vi "Approach_VUW.vi"(7 "Computer called (T/F)":bool) -> ()   [LabVIEW 2023]
uses:
  Sub_Vi/TypeDefsControls/Zposition.ctl
  Sub_Vi/TypeDefsControls/Piezo Velocity.ctl
  Sub_Vi/TypeDefsControls/Voltage.ctl
  Sub_Vi/TypeDefsControls/Xposition.ctl
  Sub_Vi/TypeDefsControls/Yposition.ctl
  Sub_Vi/TypeDefs/WayPointCluster.ctl
  Sub_Vi/TypeDefs/ChangeOnFly.ctl
  Sub_Vi/TypeDefs/Settings.ctl
  Sub_Vi/TypeDefs/Display.ctl
  Sub_Vi/TypeDefsControls/Feedback Type.ctl
  Settings.vi
panel:
  out "Current 1":cluster{"Y":dbl[], "Y":dbl[]}[](graph)
  in  "Boolean Negative":bool
  in  "Boolean Positive":bool=TRUE
  in  "Feedback Threshold (A)\nUpper":dbl
  in  "Feedback Type":T1=enum."Current 1"
  in  "Display Cluster":T2
  in  "SettingsCluster":T3={"Sample Rate (us)"=1, "Samples Per Data Point (int, power of 2)"=1000, "DistanceToBulk (um)"=-1.0, "HoldTimeScaler"=1, "SaveData"=TRUE, "DistanceToBulk (um) 2"=-1.0, "DistanceToBulk (um) 3"=-1.0}
  in  "ChangeonFly":T4
  in  "WayPointCluster":T5
  in  "Start scan Button":bool
  in  "Stop":bool
  in  "Pause":bool
  in  "Feedback Threshold (A)\nLower":dbl
  in  "Set X":bool
  in  "Set Y":bool
  in  "Y":T6=100.0 min=0.0 max=100000.0
  in  "X":T7=100.0 min=0.0 max=100000.0
  in  "Approach Voltage (V)":T8 min=-10.0 max=10.0
  in  "Approach Rate (µm/s)":T9=0.1 min=0.0
  in  "End Extension (µm)":T10 min=0.0 max=100000.0
  in  "Start Extention (µm)":T10=150.0 min=0.0 max=100000.0
  out "?":cluster{"Y":dbl[], "Y":dbl[]}[](graph)
  out "?":dbl[](graph)
  # "Settings"
  # "Pause at"
  # "Advanced Settings"
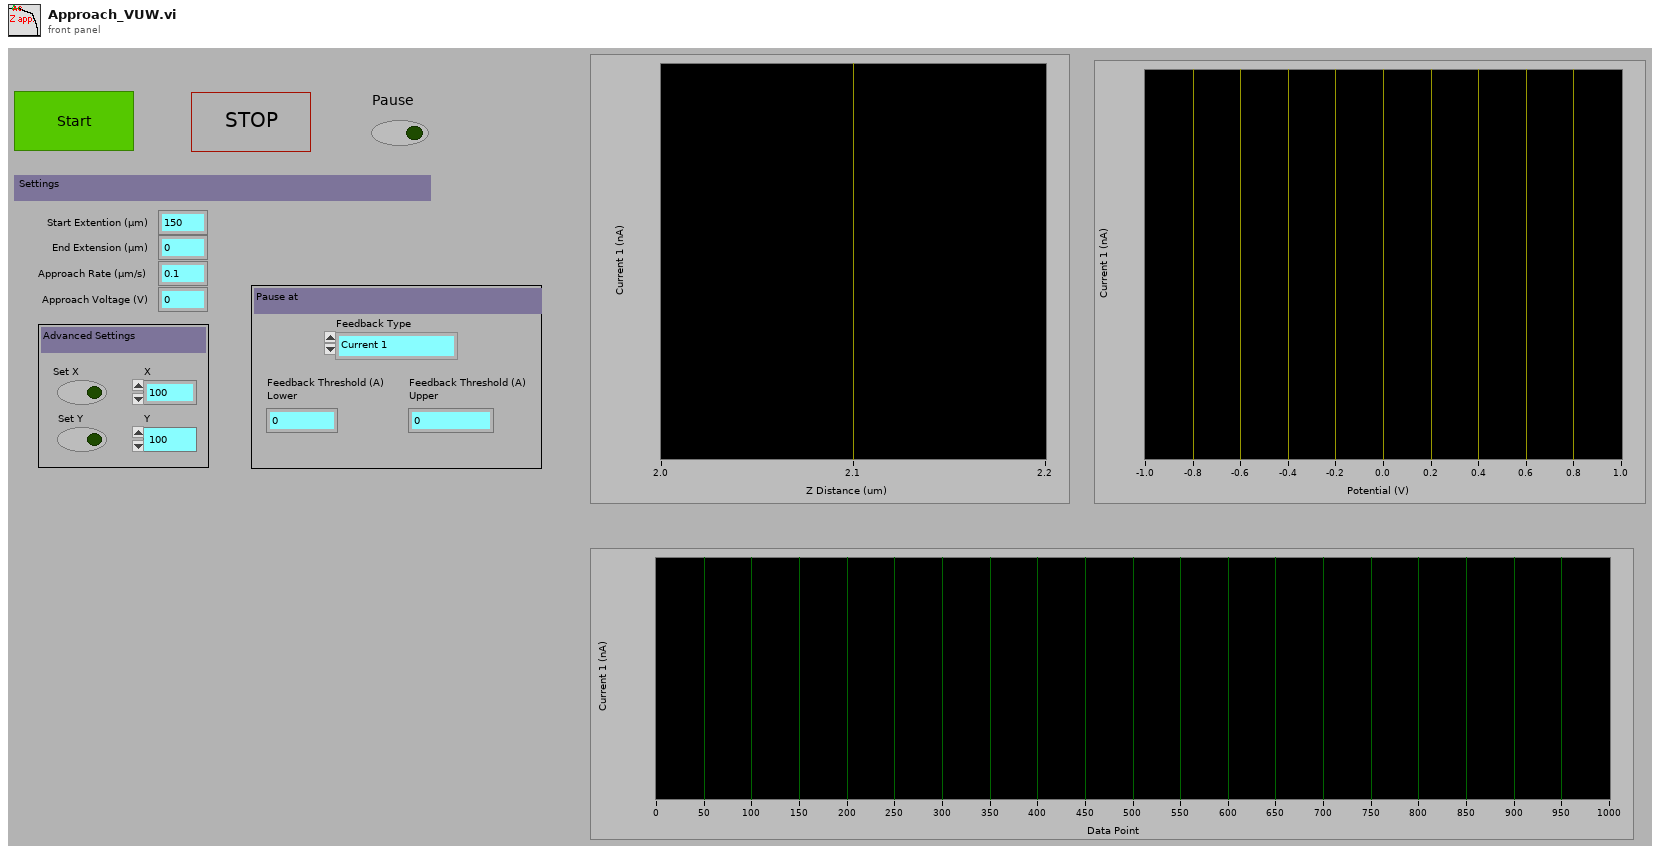
[diagram p1: front panel]
types:
  T1 = typedef "Feedback Type.ctl" = enum16{"AC Magnitude", "Current 1", "Current 2", "Phase"}
  T2 = typedef "Display.ctl" = cluster{"X":refnum<vi>, "Y":refnum<vi>, "Z":refnum<vi>, "Amp":refnum<vi>, "Phase":refnum<vi>, "t vs Z":refnum<vi>, "t vs C1":refnum<vi>, "t vs C2":refnum<vi>, "t vs C3":refnum<vi>, "t vs Amp":refnum<vi>, "t vs Phase":refnum<vi>, "t vs X":refnum<vi>, "t vs Y":refnum<vi>, "Z vs C1":refnum<vi>, "Z vs C2":refnum<vi>, "Z vs C3":refnum<vi>, "V vs C1":refnum<vi>, "V vs C2":refnum<vi>, "V vs C3":refnum<vi>, "X/Y/Z F":refnum<vi>, "X/Y/Z R":refnum<vi>, "X/Y/C1 F":refnum<vi>, "X/Y/C1 R":refnum<vi>, "X/Y/C2 F":refnum<vi>, "X/Y/C2 R":refnum<vi>, "X/Y/C3 F":refnum<vi>, "X/Y/C3 R":refnum<vi>, "NumberOfLines":u16, "um Per Pixel":dbl, "um Per Line":dbl, "X Center":dbl, "Hop X/Y/Z":refnum<vi>, "Hop X/Y/C1":refnum<vi>, "Hop X/Y/C2":refnum<vi>, "Hop X/Y/C3":refnum<vi>, "X Width":dbl, "Y Width":dbl, "Hopping Distance":dbl, "V2 vs C1":refnum<vi>, "V vs Phase":refnum<vi>, "Y Center":dbl, "Number of Pixels":dbl, "V2 vs C2":refnum<vi>, "V2 vs C3":refnum<vi>, "V vs y":refnum<vi>, "V2 vs y":refnum<vi>, "Z vs Amp":refnum<vi>, "Z vs Phase":refnum<vi>}
  T3 = typedef "Settings.ctl" = cluster{"Sample Rate (us)":u32, "Samples Per Data Point (int, power of 2)":i16, "DistanceToBulk (um)":dbl, "HoldTimeScaler":u64, "SaveData":bool, "DistanceToBulk (um) 2":dbl, "DistanceToBulk (um) 3":dbl}
  T4 = typedef "ChangeOnFly.ctl" = cluster{"Stop (boolean)":refnum<vi>, "Pause (boolean)":refnum<vi>, "EndCurrentLine (boolean)":refnum<vi>, "max movement per update step (Interger, nm)":refnum<vi>, "P (float, arb)":refnum<vi>, "Feedback set point (double, Amps)":refnum<vi>, "Voltage (double, V)":refnum<vi>, "Feedback set point 2 (double, Amps)":refnum<vi>, "Stop on Greater Than 2? (boolean)":refnum<vi>, "Stop on Greater Than? (boolean)":refnum<vi>, "Voltage 2 (double, V)":refnum<vi>, "Feedback Type (enum)":refnum<vi>, "Feedback Type 2 (enum)":refnum<vi>}
  T5 = typedef "WayPointCluster.ctl" = cluster{"X (um)":dbl[], "Y (um)":dbl[], "Z (um)":dbl[], "V (V)":dbl[], "X Velocity (um s-1)":dbl[], "Y Velocity (um s-1)":dbl[], "Z Velocity (um s-1)":dbl[], "V Velocity (V s-1)":dbl[], "FeedBack Type (enum)":u16[], "Move X (boolean)":bool[], "Move Y (boolean)":bool[], "Move Z (boolean)":bool[], "Move V (boolean)":bool[], "Jump V (boolean)":bool[], "Hold (boolean)":bool[], "Hold Time":u32[], "V2 (V)":dbl[], "Move V2":bool[], "V2 Velocity (V s-1)":dbl[], "Jump V2 (boolean)":bool[], "Update z Position delta (ms)":i16[], "Hold Feedback1":bool[], "Move Z PicoMotor":bool[], " Z PicoMotor Direction":bool[], "DIO0":bool[]}
  T6 = typedef "Yposition.ctl" = dbl
  T7 = typedef "Xposition.ctl" = dbl
  T8 = typedef "Voltage.ctl" = dbl
  T9 = typedef "Piezo Velocity.ctl" = dbl
  T10 = typedef "Zposition.ctl" = dbl
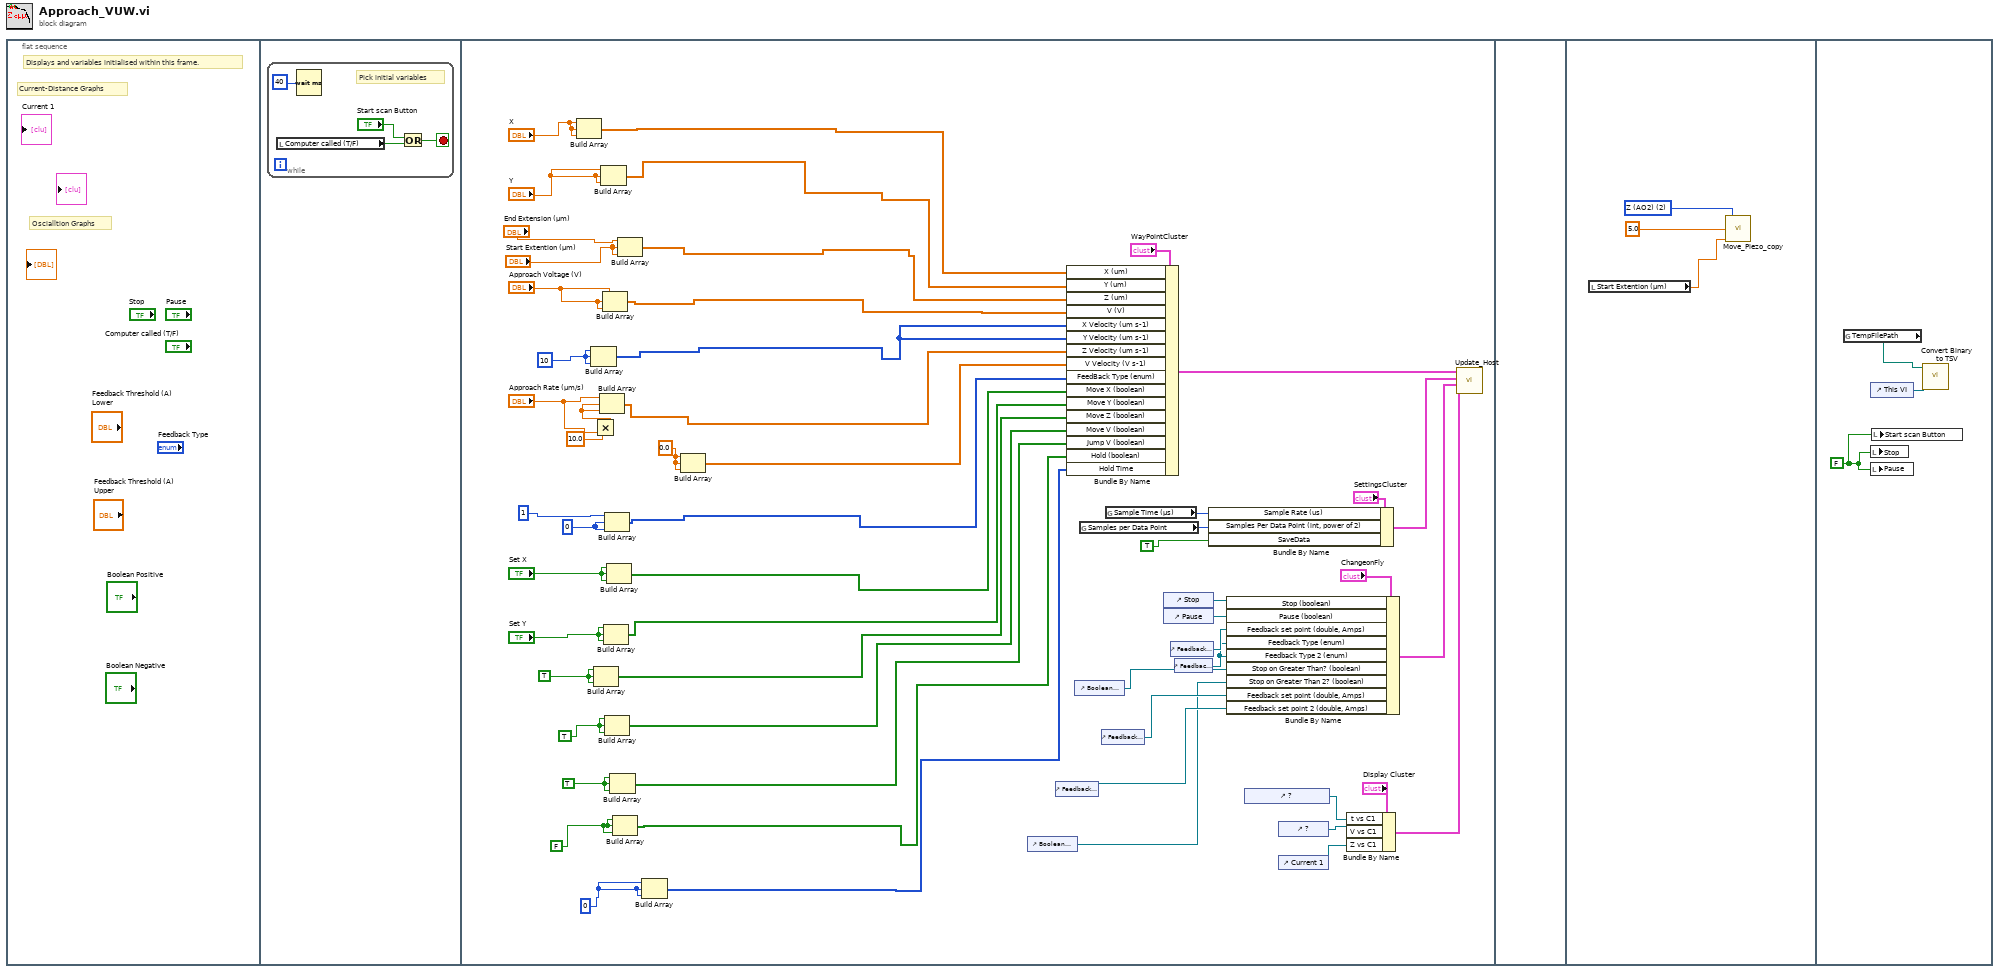
[diagram p0: block diagram]
diagram:
  n1 = flat-sequence {
    frame #0 {
      # "Oscialltion Graphs"
      # "Current-Distance Graphs"
      # "Displays and variables initialised within this frame."
    }
    frame #1 {
      n2 = while {
        stop <- w4 stop-if-true
        # "Pick initial variables"
        n3 = local read "Computer called (T/F)"() -> (w2:bool)
        n4 = Wait (ms)(milliseconds to wait=u32 40) -> ()  [unwired: 1 out]
        n5 = Or(x="Start scan Button", y=w2) -> (x .or. y?=w4:bool)
      }
    }
    frame #2 {
      w20 = u32 0 ("element")
      w18 = TRUE ("Set Z")
      w17 = TRUE ("element")
      w13 = u16 0 ("element")
      w12 = 0.0
      w19 = FALSE ("Set Z")
      w16 = TRUE ("Set Z")
      w9 = 10
      n6 = Build Array("X", "X", "X") -> (w37:T7[])
      n7 = Build Array(w9, w9, w9) -> (w32:i32[])
      n8 = Multiply(x=T9 10.0, y="Approach Rate (µm/s)") -> (x*y=w10:T9)
      n9 = Build Array(w16, w16, w16) -> (w25:bool[])
      n10 = Build Array("Approach Rate (µm/s)", w10, w10) -> (w31:T9[])
      n11 = Build Array("Y", "Y", "Y") -> (w36:T6[])
      n12 = Build Array("Approach Voltage (V)", "Approach Voltage (V)", "Approach Voltage (V)") -> (w33:T8[])
      n13 = Build Array("Set Y", "Set Y", "Set Y") -> (w26:bool[])
      n14 = Build Array(u16 1 ("Approach Type"), w13, w13) -> (w29:u16[])
      n15 = Build Array(w17, w17, w17) -> (w24:bool[])
      n16 = Build Array("Set X", "Set X", "Set X") -> (w27:bool[])
      n17 = Build Array(w18, w18, w18) -> (w23:bool[])
      n18 = Build Array(w19, w19, w19) -> (w22:bool[])
      n19 = Build Array("End Extension (µm)", "Start Extention (µm)", "Start Extention (µm)") -> (w34:T10[])
      n20 = Build Array(w20, w20, w20) -> (w21:u32[])
      n21 = Build Array(w12, w12, w12) -> (w30:dbl[])
      n22 = control-ref of="Boolean Negative"() -> (w39:refnum<vi>)
      n23 = control-ref of="Feedback Threshold (A)\nUpper"() -> (w41:refnum<vi>)
      n24 = Bundle By Name(cluster="WayPointCluster", "X (um)"=w37, "Y (um)"=w36, "Z (um)"=w34, "V (V)"=w33, "X Velocity (um s-1)"=w32, "Y Velocity (um s-1)"=w32, "Z Velocity (um s-1)"=w31, "V Velocity (V s-1)"=w30, "FeedBack Type (enum)"=w29, "Move X (boolean)"=w27, "Move Y (boolean)"=w26, "Move Z (boolean)"=w25, "Move V (boolean)"=w24, "Jump V (boolean)"=w23, "Hold (boolean)"=w22, "Hold Time"=w21) -> (w60:T5)
      n25 = control-ref of="Boolean Positive"() -> (w40:refnum<vi>)
      n26 = global read "Settings.vi" "Samples per Data Point"() -> (w51:u16)
      n27 = control-ref of="Feedback Threshold (A)\nLower"() -> (w42:refnum<vi>)
      n28 = global read "Settings.vi" "Sample Time (µs)"() -> (w52:u32)
      n29 = control-ref of="Stop"() -> (w56:refnum<vi>)
      n30 = control-ref of="Pause"() -> (w55:refnum<vi>)
      n31 = control-ref of="Feedback Threshold (A)\nLower"() -> (w46:refnum<vi>)
      n32 = control-ref of="Feedback Type"() -> (w43:refnum<vi>)
      n33 = Bundle By Name(cluster="SettingsCluster", "Sample Rate (us)"=w52, "Samples Per Data Point (int, power of 2)"=w51, "SaveData"=TRUE) -> (w58:T3)
      n34 = Bundle By Name(cluster="ChangeonFly", "Stop (boolean)"=w56, "Pause (boolean)"=w55, "Feedback set point (double, Amps)"=w46, "Feedback Type (enum)"=w43, "Feedback Type 2 (enum)"=w43, "Stop on Greater Than? (boolean)"=w40, "Stop on Greater Than 2? (boolean)"=w39, "Feedback set point (double, Amps)"=w42, "Feedback set point 2 (double, Amps)"=w41) -> (w57:T4)
      n35 = control-ref of="?"() -> (w38:refnum<vi>)
      n36 = control-ref of="?"() -> (w50:refnum<vi>)
      n37 = control-ref of="Current 1"() -> (w49:refnum<vi>)
      n38 = Bundle By Name(cluster="Display Cluster", "t vs C1"=w38, "V vs C1"=w50, "Z vs C1"=w49) -> (w59:T2)
      n39 = call "Update_Host.vi"("Display Cluster"=w59, "ChangeonFly"=w57, "SettingsCluster"=w58, "WayPointCluster"=w60) -> ()  [unwired: 6 in]
    }
    frame #3 {
    }
    frame #4 {
      w63 = u16 2 items=["X (AO0)", "Y (AO1)", "Z (AO2)", "V (AO3)", "V2 (AO4)"] ("Piezo")
      n40 = local read "Start Extention (µm)"() -> (w61:T10)
      n41 = call "Move_Piezo_copy.vi"("Piezo"=w63, "Movement Speed (µm/s)"=5.0 ("Scan Rate (um/s)"), "Position (µm) (or V)"=w61) -> ()  [unwired: 13 in]
    }
    frame #5 {
      w65 = FALSE ("Start Scanning Button")
      n42 = global read "Settings.vi" "TempFilePath"() -> (w64:path)
      n43 = control-ref of="This VI"() -> (w66:refnum<vi>)
      n44 = local write "Stop"(w65) -> ()
      n45 = local write "Pause"(w65) -> ()
      n46 = local write "Start scan Button"(w65) -> ()
      n47 = call "Convert Binary to TSV.vi"("This VI"=w66, "TDMS DataFile Name"=w64) -> ()  [unwired: 10 in]
    }
  }
